vi "mod_IQ Impairments Gain Imbalance.vi"(0 "Input Complex Waveform":T1 {"Y" format="%.3f"; "dt" format="%^.2e"; "t0" format="%.4f"}, 2 "IQ Gain Imbalance, dB":dbl format="%.2f", 11 "error in (no error)":errorcluster) -> (4 "Output Complex Waveform":T1 {"Y" format="%.3f"; "dt" format="%^.2e"; "t0" format="%.4f"}, 15 "error out":errorcluster)   [LabVIEW 2020, in "niDMT.lvlib"]
doc: "Performs the Gain Imbalance operation for IQ Impairment of an Input Data Waveform."
uses:
  <vilib>/addons/Modulation/niDMT.lvlib
  <vilib>/addons/Modulation/Analog/controls/Complex Data Waveform.ctl
  <vilib>/Analysis/5stat.llb/RMS (DBL).vi
  <vilib>/Analysis/NI_AALPro.lvlib
  <vilib>/addons/Modulation/niAMT.lvlib
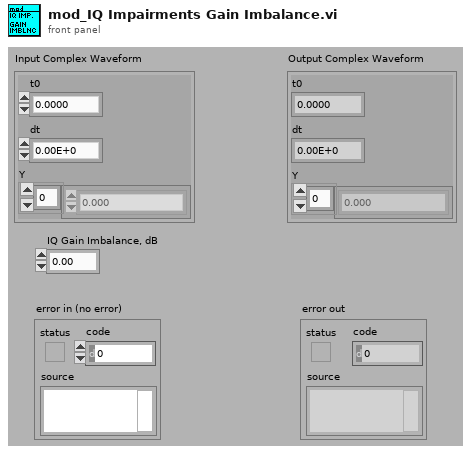
[diagram p1: front panel]
types:
  T1 = typedef "niAMT.lvlib/Complex Data Waveform.ctl" = cluster{"t0":dbl, "dt":dbl, "Y":cdb[]}
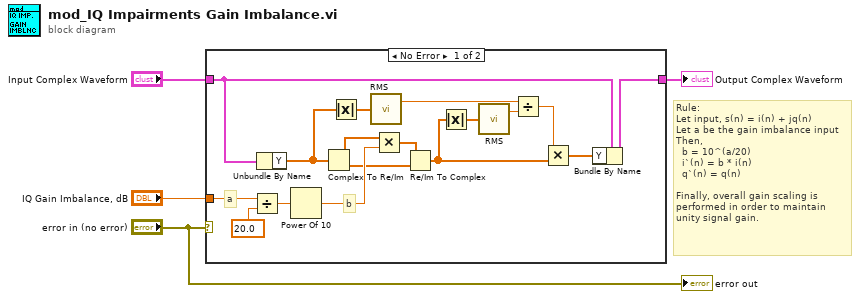
[diagram p0: block diagram]
diagram:
  # "Rule:\nLet input, s(n) = i(n) + jq(n)\nLet a be the gain imbalance input\nThen,\n  b = 10^(a/20)\n  i`(n) = b * i(n)\n  q`(n) = q(n)\n\nFinally, overall gain scaling is\nperformed in order to maintain\nunity signal gain."
  n1 = case shown="No Error" "error in (no error)" {
    tunnel: "IQ Gain Imbalance, dB" -> [w15 _]
    tunnel: "Input Complex Waveform" -> [w17 w22]
    tunnel: [w16 w22] -> w1
    frame No Error {
      # "a"
      # "b"
      n2 = Divide(x=w15, y=20.0) -> (x/y=w20:dbl)
      n3 = Unbundle By Name(w17) -> ("Y"=w13:cdb[])
      n4 = Power Of 10(x=w20) -> (10^x=w6:dbl)
      n5 = Complex To Re/Im(x + iy=w13) -> (x=w19:dbl[], y=w5:dbl[])
      n6 = Absolute Value(x=w13) -> (abs(x)=w14:dbl[])
      n7 = call-poly <vilib>:"RMS.vi"("X"=w14) -> ("rms value"=w9:dbl)  [unwired: 1 out]
      n8 = Multiply(x=w19, y=w6) -> (x*y=w18:dbl[])
      n9 = Re/Im To Complex(1:w5, 2:w18) -> (0:w11:cdb[])
      n10 = Absolute Value(x=w11) -> (abs(x)=w12:dbl[])
      n11 = call-poly <vilib>:"RMS.vi"("X"=w12) -> ("rms value"=w10:dbl)  [unwired: 1 out]
      n12 = Divide(x=w9, y=w10) -> (x/y=w7:dbl)
      n13 = Multiply(x=w7, y=w11) -> (x*y=w8:cdb[])
      n14 = Bundle By Name(cluster=w17, "Y"=w8) -> (w16:T1)
    }
    frame Error {
    }
  }
  "Output Complex Waveform" <- w1
  "error out" <- "error in (no error)"
